vi "BK Precision 5491B Configure and Run Limit Operation.vi"() -> ()   [LabVIEW 2014]
doc: "This example shows how to configure and run limit operation for pass/fail testing."
uses:
  <instrlib>/BK Precision 5491B/BK Precision 5491B.lvlib
panel:
  in  "stop":bool
  out "Limit Status":i32
  in  "Lower Limit (-1)":dbl=-1.0 format="%.3f"
  in  "Enable Limit Operation (T:Enable)":bool=TRUE
  in  "Upper Limit (1)":dbl=1.0 format="%.3f"
  in  "Serial Configuration":T1={"Baud Rate"=9600, "Parity"=0, "Data Bits"=8, "Stop Bits"=10, "Flow Control"=0} {"Flow Control" items=["None", "XON/XOFF", "RTS/CTS", "XON/XOFF & RTS/CTS", "DTR/DSR", "XON/XOFF & DTR/DSR"]; "Stop Bits" items=["1.0"=10, "1.5"=15, "2.0"=20]; "Data Bits" items=["8"=8]; "Parity" items=["None", "Odd", "Even", "Mark", "Space"]; "Baud Rate" items=["300"=300, "600"=600, "1200"=1200, "2400"=2400, "4800"=4800, "9600"=9600, "19200"=19200]}
  in  "VISA resource name":refnum<visa-resource-name>
  # "(c) 2016 B&K Precision Corporation.  ALL RIGHTS RESERVED."
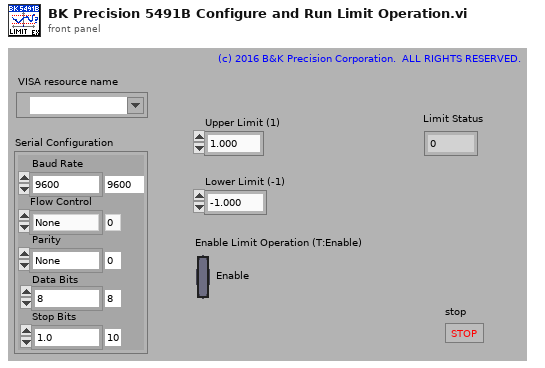
[diagram p1: front panel]
types:
  T1 = cluster{"Baud Rate":u32, "Parity":u16, "Data Bits":u16, "Stop Bits":u16, "Flow Control":u16}
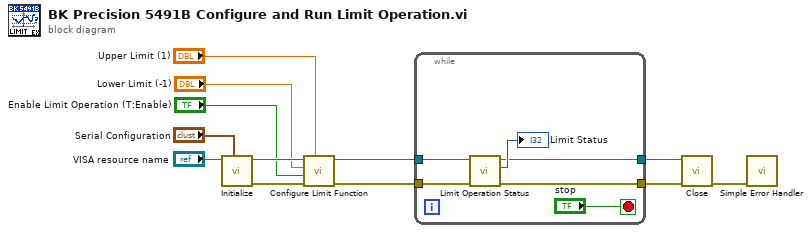
[diagram p0: block diagram]
diagram:
  n1 = call <instrlib>:"Initialize.vi"("Serial Configuration"="Serial Configuration", "VISA resource name"="VISA resource name") -> ("error out"=w8:errorcluster, "VISA resource name out"=w9:refnum<visa-resource-name>)  [unwired: 8 in]
  n2 = call <instrlib>:"Configure Limit Function.vi"("Upper Limit (1)"="Upper Limit (1)", "error in (no error)"=w8, "Enable Limit Operation (T:Enable)"="Enable Limit Operation (T:Enable)", "Lower Limit (-1)"="Lower Limit (-1)", "VISA resource name"=w9) -> ("error out"=w3:errorcluster, "VISA resource name out"=w4:refnum<visa-resource-name>)  [unwired: 5 in]
  n3 = while {
    tunnel: w4 -> [w16]
    tunnel: w3 -> [w15]
    tunnel: [w14] -> w1
    tunnel: [w13] -> w2
    stop <- "stop" stop-if-true
    n4 = call <instrlib>:"Limit Operation Status.vi"("error in (no error)"=w15, "VISA resource name"=w16) -> ("error out"=w13:errorcluster, "Limit Status"=→"Limit Status":i32, "VISA resource name out"=w14:refnum<visa-resource-name>)  [unwired: 7 in]
  }
  n5 = call <instrlib>:"Close.vi"("error in (no error)"=w2, "VISA resource name"=w1) -> ("error out"=w11:errorcluster)  [unwired: 9 in]
  n6 = call <vilib>:"Simple Error Handler.vi"("error in (no error)"=w11) -> ()  [unwired: 4 in, 5 out]
